vi "S2C_CMD_FindCmdTypes.vi"(8 "Error In":errorcluster, 11 "Command":string) -> (0 "Error Out":errorcluster, 2 "AllCmds":string[](array[string]), 3 "Types":string[](array[string]))   [LabVIEW 2015]
doc: "Finds the input types associated with a command."
uses:
  S2C_CMD_Globals.vi
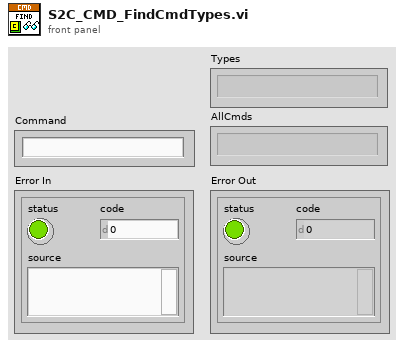
[diagram p1: front panel]
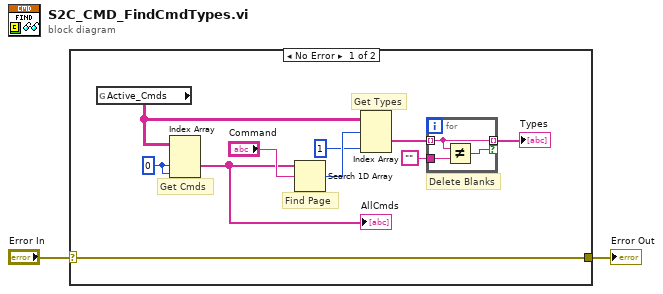
[diagram p0: block diagram]
diagram:
  n1 = case shown="No Error" "Error In" {
    selector: "Error In" -> [w7 w16]
    tunnel: [w7 w16] -> w1
    frame No Error {
      w12 = 0 ("disabled index (row)")
      # "Delete Blanks"
      # "Get Types"
      # "Find Page"
      # "Get Cmds"
      n2 = global read "S2C_CMD_Globals.vi" "Active_Cmds"() -> (w10:string[][][])
      n3 = Index Array(array=w10, index (dim 1)=w12, index (dim 2)=w12) -> (element=w6:string[])  [unwired: 1 in]
      "AllCmds" <- w6
      n4 = Search 1D Array(1D array=w6, element="Command") -> (index of element=w9:i32)  [unwired: 1 in]
      n5 = Index Array(array=w10, index (dim 0)=w9, index (dim 2)=1 ("disabled index (col)")) -> (element=w5:string[])  [unwired: 1 in]
      n6 = for {
        tunnel: w5 -> [w13] mode=indexing
        tunnel: [w13] -> w3 mode=indexing if=w15
        tunnel: "" -> [w14]
        n7 = Not Equal?(x=w13, y=w14) -> (x != y?=w15:bool)
      }
      "Types" <- w3
    }
    frame Error {
    }
  }
  "Error Out" <- w1
